vi "PWM_Lenkung_Array.vi"(9 "vorne links":dbl, 10 "vorne rechts":dbl) -> (0 "16 IR true":bool, 2 "PWM Lenkung":dbl, 3 "Linefollow_Array":bool[](array[boolean]))   [LabVIEW 2016]
doc: "VI berrechnet Abweichung des Linearray zur Mittellinie\n05.04.17_Tloe"
uses:
  <vilib>/myRIO/Instrument Drivers/Onboard IO/DIO/typedefs/DIO Reference.ctl
  <vilib>/myRIO/Common/Instrument Driver Framework/Utilities/typedefs/myRIO Generic Hardware Reference.ctl
  <vilib>/myRIO/Common/Instrument Driver Framework/Utilities/typedefs/Hardware Version Enum.ctl
  <vilib>/myRIO/Common/Instrument Driver Framework/Utilities/typedefs/myRIO v1.0 Reference.ctl
  <vilib>/myRIO/Common/Instrument Driver Framework/Utilities/typedefs/Generic FPGA Reference.ctl
  <vilib>/myRIO/Common/Instrument Driver Framework/myRIO v1.0/DIO/typedefs/DIO Channels List.ctl
  <vilib>/myRIO/Common/Instrument Driver Framework/myRIO v1.0/DIO/typedefs/DIO Channels Enum.ctl
  <vilib>/userdefined/High Color/nirio_resource_hc.ctl
  <vilib>/myRIO/Common/Instrument Driver Framework/Utilities/vis/Is FPGA Ref Available.vi
  <vilib>/myRIO/Common/Instrument Driver Framework/myRIO v1.0/DIO/vis/myRIO v1.1 Open DIO.vi
  <vilib>/myRIO/Instrument Drivers/Onboard IO/DIO/vis/Read.vi
  <vilib>/myRIO/Common/Instrument Driver Framework/Utilities/vis/Validate Channels.vi
  <vilib>/myRIO/Common/Instrument Driver Framework/myRIO v1.0/DIO/vis/myRIO v1.0 Reserve DIO.vi
  <vilib>/myRIO/Common/Instrument Driver Framework/myRIO v1.0/Resource Manager/vis/myRIO v1.0 Reserve Channel List.vi
  <vilib>/myRIO/Common/Instrument Driver Framework/myRIO v1.0/DIO/vis/myRIO v1.0 Build MUX Configuration DIO.vi
  <vilib>/myRIO/Common/Instrument Driver Framework/myRIO v1.0/Resource Manager/vis/myRIO v1.0 Reserve Channel.vi
  <vilib>/myRIO/Common/Instrument Driver Framework/myRIO v1.0/Resource Manager/vis/myRIO v1.0 Unreserve Channel.vi
  <vilib>/myRIO/Common/Instrument Driver Framework/myRIO v1.0/Resource Manager/vis/myRIO v1.0 Create Configuration List.vi
  <vilib>/myRIO/Common/Instrument Driver Framework/myRIO v1.0/Resource Manager/vis/myRIO v1.0 Build Mutex Name.vi
  <vilib>/Utility/VariantDataType/GetNumericInfo.vi
  <vilib>/Utility/error.llb/Error Cluster From Error Code.vi
  <vilib>/myRIO/Common/Instrument Driver Framework/myRIO v1.0/myRIO v1.1 Open.vi
  <vilib>/myRIO/Common/Instrument Driver Framework/Utilities/vis/IO Manager.vi
  <vilib>/myRIO/Common/Instrument Driver Framework/Utilities/vis/Configuration Manager.vi
  <vilib>/myRIO/Common/Instrument Driver Framework/myRIO v1.0/Resource Manager/vis/myRIO v1.0 Configure IO.vi
  <vilib>/myRIO/Common/Instrument Driver Framework/myRIO v1.0/myRIO v1.0 Close.vi
  <vilib>/myRIO/Common/Instrument Driver Framework/myRIO v1.0/DIO/vis/myRIO v1.0 Read DIO.vi
  <vilib>/addons/control/pid/pid.llb/PID (DBL).vi
  <vilib>/myRIO/Express VI/Onboard IO/DI/DI Express VI.xnode
  <vilib>/myRIO/Instrument Drivers/Onboard IO/DIO/vis/myRIO DIO Open.xnode
  <vilib>/myRIO/Instrument Drivers/Onboard IO/DIO/DIO.lvlib
  <vilib>/addons/control/pid/NI_PID_pid.lvlib
panel:
  in  "PID IR":T1={"proportional gain (Kc)"=0.5, "integral time (Ti, min)"=1.0, "derivative time (Td, min)"=0.001} {"proportional gain (Kc)" format="%#_10g"; "integral time (Ti, min)" format="%#_10g"; "derivative time (Td, min)" format="%#_10g"}
  in  "PID Array":T1={"proportional gain (Kc)"=0.61, "integral time (Ti, min)"=0.08, "derivative time (Td, min)"=0.32}
  in  "Sensorarray\nZusatzwerte":dbl[](array[numeric])=[8.0, 7.0, 6.0, 5.0, 4.0, 3.0, 2.0, 1.0, -1.0, -2.0, -3.0, -4.0, -5.0, -6.0, -7.0, -8.0]
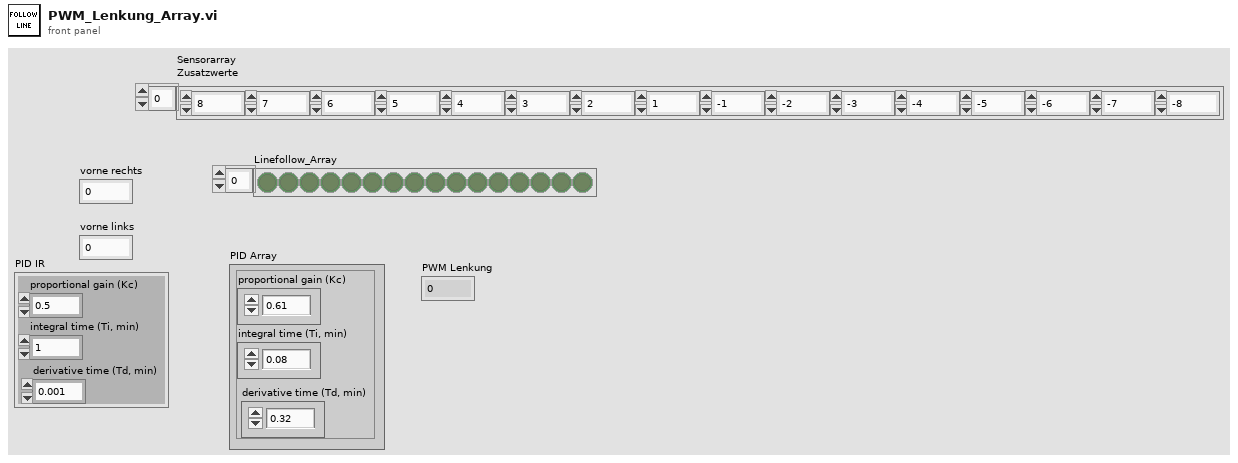
[diagram p1: front panel]
types:
  T1 = cluster{"proportional gain (Kc)":dbl, "integral time (Ti, min)":dbl, "derivative time (Td, min)":dbl}
  T2 = cluster{"A/DIO0 (Pin 11)":bool, "A/DIO1 (Pin 13)":bool, "A/DIO2 (Pin 15)":bool, "A/DIO3 (Pin 17)":bool, "A/DIO4 (Pin 19)":bool, "A/DIO5 (Pin 21)":bool, "A/DIO6 (Pin 23)":bool, "A/DIO7 (Pin 25)":bool, "B/DIO7 (Pin 25)":bool, "B/DIO6 (Pin 23)":bool, "B/DIO5 (Pin 21)":bool, "B/DIO3 (Pin 17)":bool, "B/DIO4 (Pin 19)":bool, "B/DIO2 (Pin 15)":bool, "B/DIO1 (Pin 13)":bool, "B/DIO12 (Pin 22)":bool}
  T3 = cluster{"A/DIO0 (Pin 11)":i16, "A/DIO1 (Pin 13)":i16, "A/DIO2 (Pin 15)":i16, "A/DIO3 (Pin 17)":i16, "A/DIO4 (Pin 19)":i16, "A/DIO5 (Pin 21)":i16, "A/DIO6 (Pin 23)":i16, "A/DIO7 (Pin 25)":i16, "B/DIO7 (Pin 25)":i16, "B/DIO6 (Pin 23)":i16, "B/DIO5 (Pin 21)":i16, "B/DIO3 (Pin 17)":i16, "B/DIO4 (Pin 19)":i16, "B/DIO2 (Pin 15)":i16, "B/DIO1 (Pin 13)":i16, "B/DIO12 (Pin 22)":i16}
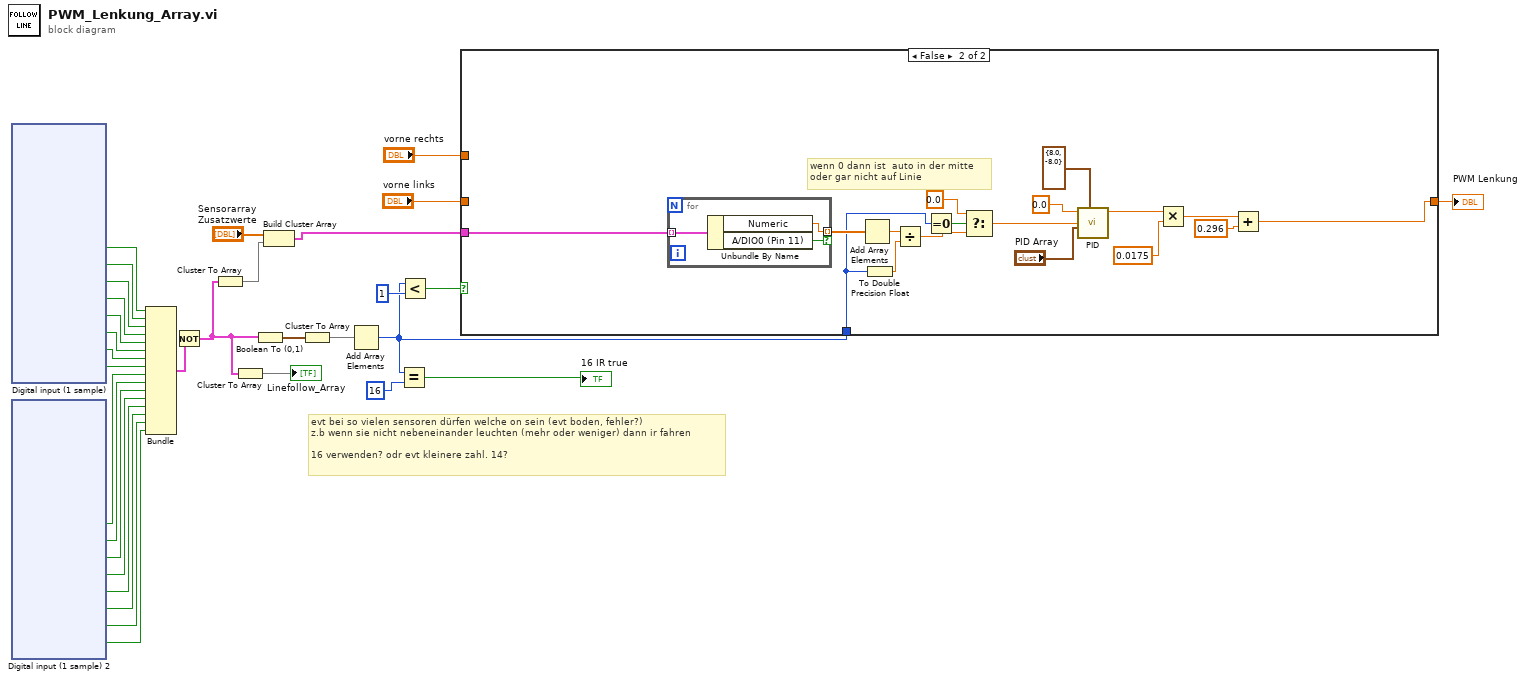
[diagram p0: block diagram]
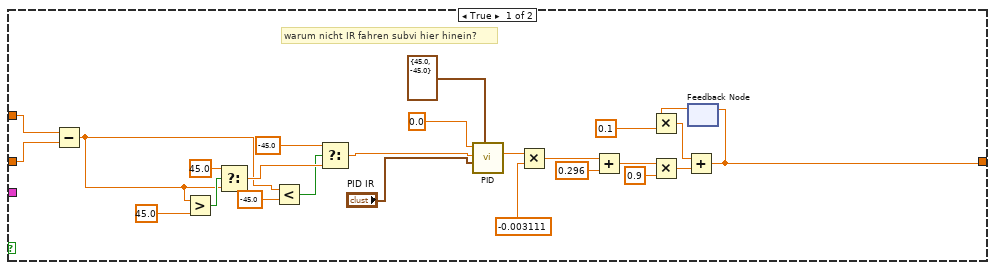
[diagram p2: hidden frame]
diagram:
  # "evt bei so vielen sensoren dürfen welche on sein (evt boden, fehler?)\nz.b wenn sie nicht nebeneinander leuchten (mehr oder weniger) dann ir fahren\n\n16 verwenden? odr evt kleinere zahl. 14?"
  n1 = xnode "Digital input (1 sample)"() -> ("A/DIO0 (Pin 11)"=w23:bool, "A/DIO1 (Pin 13)"=w24:bool, "A/DIO2 (Pin 15)"=w25:bool, "A/DIO3 (Pin 17)"=w26:bool, "A/DIO4 (Pin 19)"=w27:bool, "A/DIO5 (Pin 21)"=w28:bool, "A/DIO6 (Pin 23)"=w29:bool, "A/DIO7 (Pin 25)"=w30:bool)  [unwired: 1 in, 1 out]
  n2 = xnode "Digital input (1 sample) 2"() -> ("B/DIO7 (Pin 25)"=w8:bool, "B/DIO6 (Pin 23)"=w7:bool, "B/DIO5 (Pin 21)"=w6:bool, "B/DIO3 (Pin 17)"=w5:bool, "B/DIO4 (Pin 19)"=w4:bool, "B/DIO2 (Pin 15)"=w3:bool, "B/DIO1 (Pin 13)"=w2:bool, "B/DIO12 (Pin 22)"=w1:bool)  [unwired: 1 in, 1 out]
  n3 = Bundle("A/DIO0 (Pin 11)"=w23, "A/DIO1 (Pin 13)"=w24, "A/DIO2 (Pin 15)"=w25, "A/DIO3 (Pin 17)"=w26, "A/DIO4 (Pin 19)"=w27, "A/DIO5 (Pin 21)"=w28, "A/DIO6 (Pin 23)"=w29, "A/DIO7 (Pin 25)"=w30, "B/DIO7 (Pin 25)"=w8, "B/DIO6 (Pin 23)"=w7, "B/DIO5 (Pin 21)"=w6, "B/DIO3 (Pin 17)"=w5, "B/DIO4 (Pin 19)"=w4, "B/DIO2 (Pin 15)"=w3, "B/DIO1 (Pin 13)"=w2, "B/DIO12 (Pin 22)"=w1) -> (w22:T2)  [unwired: 1 in]
  n4 = Not(x=w22) -> (.not. x?=w15:T2)
  n5 = Cluster To Array(cluster=w15) -> (array=w17:bool[])
  n6 = Cluster To Array(cluster=w15) -> (array=→"Linefollow_Array":bool[])
  n7 = Boolean To (0,1)(Boolean=w15) -> (0, 1=w31:T3)
  n8 = Build Cluster Array("Sensorarray\nZusatzwerte", w17) -> (w12:cluster{"Numeric":dbl, "A/DIO0 (Pin 11)":bool}[])
  n9 = Cluster To Array(cluster=w31) -> (array=w14:i16[])
  n10 = Add Array Elements(numeric array=w14) -> (sum=w11:i16)
  n11 = Equal?(x=w11, y=i16 16) -> (x = y?=→"16 IR true":bool)
  n12 = Less?(x=w11, y=i16 1) -> (x < y?=w13:bool)
  n13 = case shown="False" w13 {
    tunnel: [w34 w60] -> w18
    tunnel: w12 -> [_ w59]
    tunnel: w11 -> [_ w58]
    tunnel: "vorne rechts" -> [w39 _]
    tunnel: "vorne links" -> [w38 _]
    frame True {
      # "warum nicht IR fahren subvi hier hinein?"
      n14 = Subtract(x=w39, y=w38) -> (x-y=w41:dbl)
      n15 = Greater?(x=w41, y=45.0) -> (0:w48:bool)
      n16 = Select(t=45.0, s=w48, f=w41) -> (s? t:f=w43:dbl)
      n17 = Less?(x=w41, y=-45.0) -> (x < y?=w33:bool)
      n18 = Select(t=-45.0, s=w33, f=w43) -> (s? t:f=w42:dbl)
      n19 = call-poly <vilib>:"PID.vi"("output range"=cluster{"output high":dbl, "output low":dbl} {"output high"=45.0, "output low"=-45.0}, "PID gains"="PID IR", "process variable"=w42, "setpoint"=0.0) -> ("output"=w57:dbl)  [unwired: 6 in, 1 out]
      n20 = Multiply(x=w57, y=-0.003111) -> (x*y=w54:dbl)
      n21 = Add(x=w54, y=0.296) -> (x+y=w56:dbl)
      n22 = Multiply(x=w56, y=0.9) -> (x*y=w52:dbl)
      n23 = feedback #1() -> (w35:dbl)  [unwired: 1 in]
      n24 = Multiply(x=w35, y=0.1) -> (x*y=w51:dbl)
      n25 = Add(x=w51, y=w52) -> (x+y=w34:dbl)
      n26 = feedback-in #1(w34) -> ()
    }
    frame False {
      # "wenn 0 dann ist  auto in der mitte \noder gar nicht auf Linie"
      n27 = for {
        tunnel: [w77] -> w72 mode=indexing if=w76
        tunnel: w59 -> [w75] mode=indexing
        n28 = Unbundle By Name(w75) -> ("Numeric"=w77:dbl, "A/DIO0 (Pin 11)"=w76:bool)
      }
      n29 = Add Array Elements(numeric array=w72) -> (sum=w73:dbl)
      n30 = To Double Precision Float(number=w58) -> (double precision float=w74:dbl)
      n31 = Divide(x=w73, y=w74) -> (x/y=w71:dbl)
      n32 = Equal To 0?(x=w58) -> (x = 0?=w69:bool)
      n33 = Select(t=0.0, s=w69, f=w71) -> (s? t:f=w61:dbl)
      n34 = call-poly <vilib>:"PID.vi"("output range"=cluster{"output high":dbl, "output low":dbl} {"output high"=8.0, "output low"=-8.0}, "PID gains"="PID Array", "process variable"=w61, "setpoint"=0.0) -> ("output"=w66:dbl)  [unwired: 6 in, 1 out]
      n35 = Multiply(x=w66, y=0.0175) -> (x*y=w67:dbl)
      n36 = Add(x=w67, y=0.296) -> (x+y=w60:dbl)
    }
  }
  "PWM Lenkung" <- w18
